vi "saveAccelerationTimeDataToTDMS.vi"(8 "ErrorIn":errorcluster, 11 "QueuesIn":T1) -> (0 "ErrorOut":errorcluster, 3 "QueuesOut":T1)   [LabVIEW 2019]
uses:
  utilities/Queues.ctl
  MobileAnalyzer/mainVIs/UIVIs/AccelerationDataFrames.ctl
  GUIVIs/GUIOutput.ctl
  masterVIs/Command.ctl
  saveAccelerationTimeDataToTDMSVIs/saveAccelerationTimeDataToTDMSState.ctl
  masterVIs/Thread.ctl
  DialogsVIs/FilePathToSaveAction.ctl
panel:
  in  "Stop":bool=TRUE
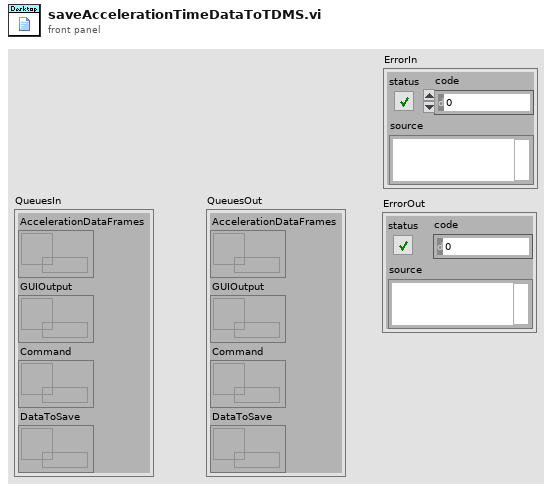
[diagram p1: front panel]
types:
  T1 = typedef "Queues.ctl" = cluster{"AccelerationDataFrames":refnum<queue>, "GUIOutput":refnum<queue>, "Command":refnum<queue>, "DataToSave":refnum<queue>}
  T2 = typedef "Thread.ctl" = enum16{"GUI", "communicateWithAnalyzer", "saveDataToTDMS"}
  T3 = typedef "saveAccelerationTimeDataToTDMSState.ctl" = enum16{"Idle", "Init", "Save to TDMS", "End"}
  T4 = typedef "Command.ctl" = enum16{"None", "Connect", "Start", "Stop", "RestartAnalyzer", "Exit", "OpenDataFile", "CanBegin", "FileToSaveSettings"}
  T5 = typedef "FilePathToSaveAction.ctl" = enum16{"Build new path", "Update index", "Get file path", "Get current settings"}
  T6 = enum16{"open", "open or create", "create or replace", "create", "open (read-only)"}
  T7 = typedef "DesktopAppSettings.ctl" = cluster{"MobileAnalyzer IP":string, "Network Stream Timeout Code":i32, "Endpoint Destroyed Code":i32, "Save to file?":bool, "All threads":T2[]}
  T8 = typedef "AccelerationDataFrames.ctl" = cluster{"AccelerationData":waveform(dbl)[], "Amplitudes":cluster{"f0":dbl, "df":dbl, "real part":dbl[]}[], "Phases":cluster{"f0":dbl, "df":dbl, "imaginary part":dbl[]}[]}
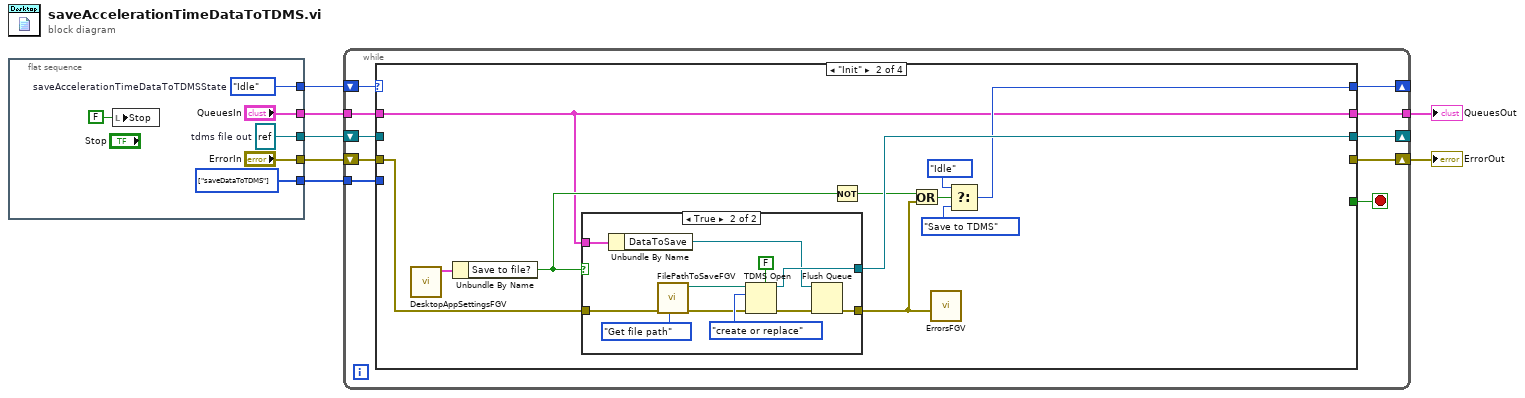
[diagram p0: block diagram]
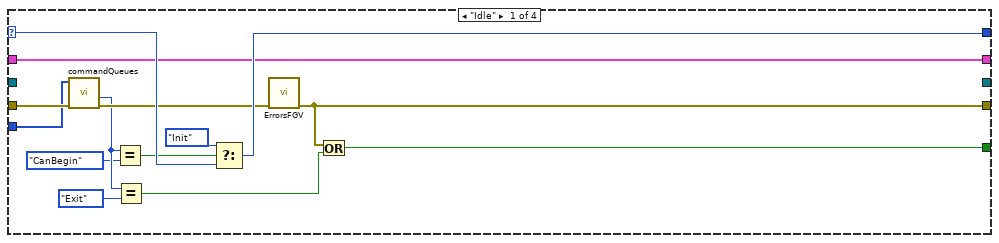
[diagram p2: hidden frame]
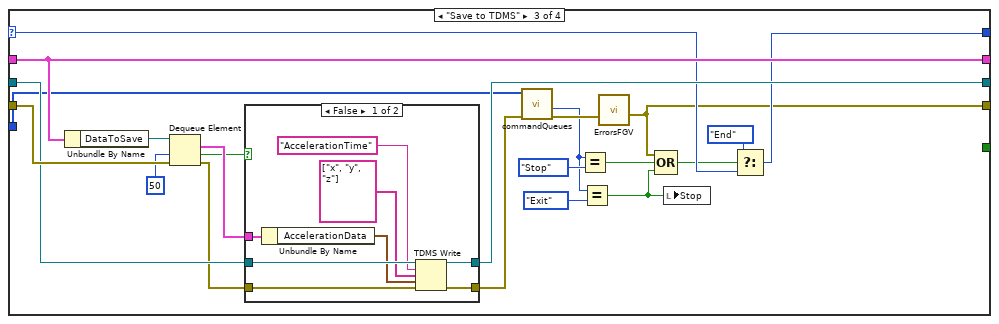
[diagram p4: hidden frame]
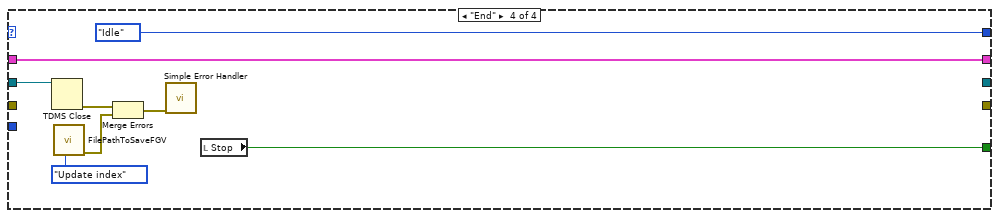
[diagram p6: hidden frame]
diagram:
  n1 = flat-sequence {
    tunnel: [w13] -> w7
    tunnel: ["ErrorIn"] -> w6
    tunnel: [w11] -> w4
    tunnel: ["QueuesIn"] -> w3
    tunnel: [w8] -> w1
    frame #0 {
      w8 = T2[] [enum."saveDataToTDMS"] items=["GUI", "communicateWithAnalyzer", "saveDataToTDMS"] ("Threads")
      w11 = refnum<k34> refnum  # tdms file out
      w13 = saveAccelerationTimeDataToTDMSState."Idle"  # saveAccelerationTimeDataToTDMSState
      n2 = local write "Stop"(FALSE ("Stop")) -> ()
    }
  }
  n3 = while {
    shift-right: [w19] -> _
    shift-left: w7 -> [w23]
    tunnel: w3 -> [w22]
    shift-right: [w16] -> w5
    shift-left: w6 -> [w21]
    tunnel: [w20] -> w2
    shift-right: [w18] -> _
    shift-left: w4 -> [w17]
    tunnel: w1 -> [w14]
    stop <- w15 stop-if-true
    n4 = case shown="\"Init\"" w23 {
      selector: w23 -> [w37 _ w73 _]
      tunnel: w22 -> [w34 w38 w82 w98]
      tunnel: w21 -> [w28 w48 w80 _]
      tunnel: [w34 w38 w82 w98] -> w20
      tunnel: [w30 _ w67 _] -> w16
      tunnel: [w35 _ _ w97] -> w15
      tunnel: [w36 w41 w71 saveAccelerationTimeDataToTDMSState."Idle" ("saveAccelerationTimeDataToTDMSState")] -> w19
      tunnel: [_ w47 w75 _] -> w18
      tunnel: w17 -> [_ _ w77 w100]
      tunnel: w14 -> [w25 _ w62 _]
      frame "Idle" {
        n5 = call "commandQueues.vi"("ErrorIn"=w28, "Threads"=w25) -> ("ErrorOut"=w27:errorcluster, "CommandOut"=w26:T4)  [unwired: 8 in]
        n6 = Equal?(x=w26, y=Command."CanBegin") -> (x = y?=w32:bool)
        n7 = Equal?(x=w26, y=Command."Exit") -> (x = y?=w29:bool)
        n8 = Select(t=saveAccelerationTimeDataToTDMSState."Init", s=w32, f=w37) -> (s? t:f=w36:T3)
        n9 = call "ErrorsFGV.vi"("CriticalErrorIn"=w27) -> ("CriticalErrorOut"=w30:errorcluster)  [unwired: 7 in, 3 out]
        n10 = Or(x=w30, y=w29) -> (x .or. y?=w35:bool)
      }
      frame "Init" {
        n11 = call "DesktopAppSettingsFGV.vi"() -> ("DesktopAppSettingsOut"=w40:T7)  [unwired: 11 in]
        n12 = Unbundle By Name(w40) -> ("Save to file?"=w45:bool)
        n13 = case shown="True" w45 {
          tunnel: w48 -> [w49 w53]
          tunnel: [w49 w54] -> w39
          tunnel: [_ w58] -> w47
          tunnel: w38 -> [_ w57]
          frame False {
          }
          frame True {
            n14 = Unbundle By Name(w57) -> ("DataToSave"=w56:refnum<queue>)
            n15 = call "FilePathToSaveFGV.vi"("FilePathToSaveAction"=FilePathToSaveAction."Get file path", "ErrorIn"=w53) -> ("ErrorOut"=w52:errorcluster, "File path"=w50:path)  [unwired: 6 in, 2 out]
            n16 = TDMS Open(5:FALSE ("create index file? (T)"), 8:w52, 10:T6."create or replace" ("operation (0:open)"), 11:w50) -> (0:w55:errorcluster, 3:w58:refnum<k34>)  [unwired: 3 in]
            n17 = Flush Queue(queue=w56, error in (no error)=w55) -> (error out=w54:errorcluster)  [unwired: 2 out]
          }
        }
        n18 = Not(x=w45) -> (.not. x?=w44:bool)
        n19 = Or(x=w44, y=w39) -> (x .or. y?=w46:bool)
        n20 = call "ErrorsFGV.vi"("InternalErrorIn"=w39) -> ()  [unwired: 7 in, 4 out]
        n21 = Select(t=saveAccelerationTimeDataToTDMSState."Idle", s=w46, f=saveAccelerationTimeDataToTDMSState."Save to TDMS" ("saveAccelerationTimeDataToTDMSState")) -> (s? t:f=w41:T3)
      }
      frame "Save to TDMS" {
        n22 = Unbundle By Name(w82) -> ("DataToSave"=w81:refnum<queue>)
        n23 = Dequeue Element(queue=w81, timeout in ms (-1)=50, error in (no error)=w80) -> (element=w78:T8, timed out?=w74:bool, error out=w76:errorcluster)  [unwired: 1 out]
        n24 = case shown="False" w74 {
          tunnel: w78 -> [w90 _]
          tunnel: w77 -> [w89 w92]
          tunnel: w76 -> [w88 w91]
          tunnel: [w85 w91] -> w63
          tunnel: [w84 w92] -> w75
          frame False {
            n25 = Unbundle By Name(w90) -> ("AccelerationData"=w83:waveform(dbl)[])
            n26 = TDMS Write(0:w89, 5:"AccelerationTime" ("group name in (Untitled)"), 7:string[] ["x", "y", "z"] ("channel name(s) in (Untitled)"), 9:w83, 11:w88) -> (4:w84:refnum<k34>, 15:w85:errorcluster)  [unwired: 1 in, 2 out]
          }
          frame True {
          }
        }
        n27 = call "commandQueues.vi"("ErrorIn"=w63, "Threads"=w62) -> ("ErrorOut"=w64:errorcluster, "CommandOut"=w61:T4)  [unwired: 8 in]
        n28 = Equal?(x=w61, y=Command."Stop") -> (x = y?=w69:bool)
        n29 = Equal?(x=w61, y=Command."Exit") -> (x = y?=w65:bool)
        n30 = call "ErrorsFGV.vi"("InternalErrorIn"=w64) -> ("InternalErrorOut"=w67:errorcluster)  [unwired: 7 in, 3 out]
        n31 = Compound Arithmetic op=OR(w67, w69, w65) -> (w66:bool)
        n32 = local write "Stop"(w65) -> ()
        n33 = Select(t=saveAccelerationTimeDataToTDMSState."End", s=w66, f=w73) -> (s? t:f=w71:T3)
      }
      frame "End" {
        n34 = TDMS Close(11:w100) -> (0:w95:errorcluster)  [unwired: 1 in, 1 out]
        n35 = call "FilePathToSaveFGV.vi"("FilePathToSaveAction"=FilePathToSaveAction."Update index") -> ("ErrorOut"=w94:errorcluster)  [unwired: 7 in, 3 out]
        n36 = Merge Errors(w95, w94) -> (w93:errorcluster)
        n37 = call <vilib>:"Simple Error Handler.vi"("error in (no error)"=w93) -> ()  [unwired: 4 in, 5 out]
        n38 = local read "Stop"() -> (w97:bool)
      }
    }
  }
  "ErrorOut" <- w5
  "QueuesOut" <- w2
